vi "Unsubscribe.vi"(8 "error in (no error)":errorcluster, 10 "SubscriptionPolicy":T1, 11 "IObserver in":refnum<class "IObserver.lvclass">) -> (0 "error out":errorcluster, 3 "IObserver out":refnum<class "IObserver.lvclass">)   [LabVIEW 2020, in "IObserver.lvlib" / "IObserver.lvclass"]
doc: "<License>\nCopyright © 2017 Composed Systems, LLC | All rights reserved\nwww.composed.io\n\nAuthor: Ethan Stern <ethan.stern@composed.io>\n\nThis software is provided \"AS IS\" WITHOUT WARRANTIES, either express or implied, AND IS FOR EDUCATIONAL PURPOSES ONLY.\n</License>"
uses:
  <vilib>/gpm_packages/@cs/mva-core/Source/IObserver/IObserver/IObserver.lvclass
  <vilib>/gpm_packages/@cs/mva-core/Source/IMediator/ISubscriptionPolicy/ISubscriptionPolicy Reference.ctl
  <vilib>/gpm_packages/@cs/mva-core/Source/IMediator/ISubscriptionPolicy/ISubscriptionPolicy.lvclass
  <vilib>/gpm_packages/@cs/mva-core/Source/IObserver/IObserver/IObserver.lvclass/IObserver.ctl
  <vilib>/gpm_packages/@cs/mva-core/Source/IMediator/IMediator Messages/Unsubscribe Msg/Unsubscribe Msg.lvclass/Unsubscribe Msg.ctl
  <vilib>/gpm_packages/@cs/actor-framework-messages/Source/RoundTripMessage/RoundTripMessage.lvclass/RoundTripMessage.ctl
  <vilib>/ActorFramework/Message Enqueuer/Message Enqueuer.lvclass/Message Enqueuer.ctl
  <vilib>/gpm_packages/@cs/actor-framework-messages/Source/RoundTripMessage/Return Round-Trip Message.vi
  <vilib>/ActorFramework/Message Enqueuer/Enqueue.vi
  <vilib>/gpm_packages/@cs/mva-core/Source/IMediator/IMediator Messages/Unsubscribe Msg/Unsubscribe Msg.lvclass
  C:/Program Files/National Instruments/LabVIEW 2020/vi.lib/gpm_packages/@cs/actor-framework-messages/Source/RoundTripMessage/RoundTripMessage.lvclass
  <vilib>/gpm_packages/@cs/actor-framework-messages/Source/RoundTripMessage/RoundTripMessage.lvclass
  C:/Program Files/National Instruments/LabVIEW 2020/vi.lib/ActorFramework/Message/Message.lvclass
  <vilib>/ActorFramework/Message Priority Queue/Priority Enqueue.vi
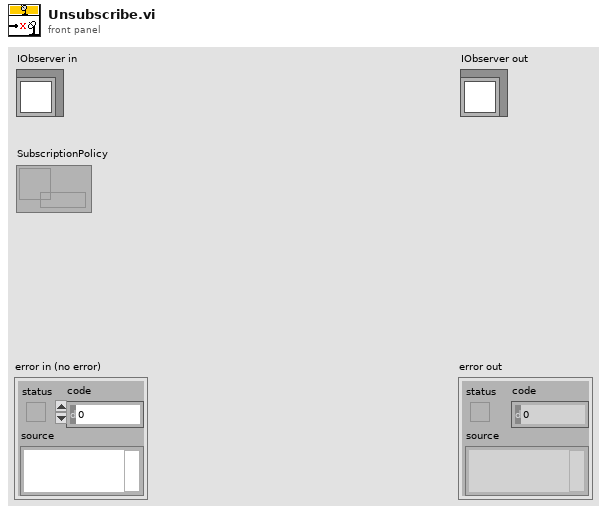
[diagram p1: front panel]
types:
  T1 = typedef "IMediator.lvlib/ISubscriptionPolicy.lvclass/ISubscriptionPolicy Reference.ctl" = refnum<data-value>
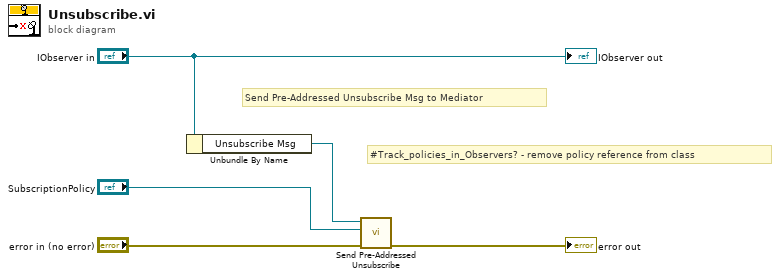
[diagram p0: block diagram]
diagram:
  # "#Track_policies_in_Observers? - remove policy reference from class"
  # "Send Pre-Addressed Unsubscribe Msg to Mediator"
  n1 = Unbundle By Name("IObserver in") -> ("Unsubscribe Msg"=w4:refnum<class "Unsubscribe Msg.lvclass">)
  n2 = call <vilib>:"Send Pre-Addressed Unsubscribe.vi"("error in (no error)"="error in (no error)", "SubscriptionPolicy"="SubscriptionPolicy", "Unsubscribe Msg In"=w4) -> ("error out"=→"error out":errorcluster)  [unwired: 8 in]
  "IObserver out" <- "IObserver in"
